vi "AddContained.vi"(8 "error in (no error)":errorcluster, 9 "Item to contain":refnum<class "ILabVIEWItem.lvclass">, 11 "CLabVIEWItemVIM in":refnum<class "CLabVIEWItemVIM.lvclass">) -> (0 "error out":errorcluster, 1 "Relationship type":T1, 3 "CLabVIEWItemVIM out":refnum<class "CLabVIEWItemVIM.lvclass">)   [LabVIEW 2020, in "LabVIEWFiles.lvlib" / "CLabVIEWItemVIM.lvclass"]
uses:
  CLabVIEWItemVIM.lvclass
  LabVIEWObjectInterfaces/ILabVIEWItem/ILabVIEWItem.lvclass
  LabVIEWObjectInterfaces/ILabVIEWItem/RelationshipType.ctl
  CLabVIEWItemVI/CLabVIEWItemVI.lvclass
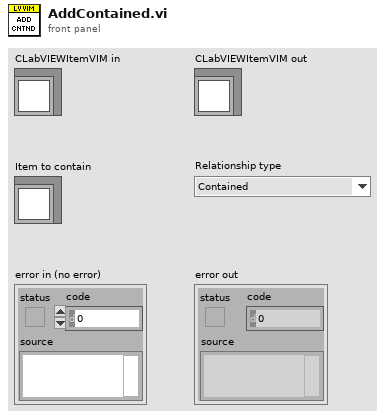
[diagram p1: front panel]
types:
  T1 = typedef "LabVIEWObjectInterfaces.lvlib/ILabVIEWItem.lvclass/RelationshipType.ctl" = enum16{"Contained", "Dependency", "Parent", "Same item", "Related", "None"}
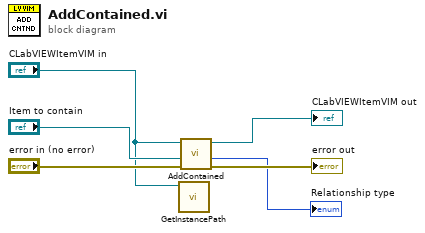
[diagram p0: block diagram]
diagram:
  n1 = call-dynamic "GetInstancePath.vi"("CLabVIEWItemVIM in"="CLabVIEWItemVIM in") -> ()  [unwired: 8 in, 3 out]
  n2 = call-parent "AddContained.vi"("error in (no error)"="error in (no error)", "Item to contain"="Item to contain", "CLabVIEWItem in"="CLabVIEWItemVIM in") -> ("error out"=→"error out":errorcluster, "Relationship type"=→"Relationship type":T1, "CLabVIEWItem out"=→"CLabVIEWItemVIM out":refnum<class "CLabVIEWItemVIM.lvclass">)  [unwired: 6 in]
